vi "SetData.vi"(8 "error in (no error)":errorcluster caption="Fehler (Eingang, kein Fehler)", 9 "Data":variant, 10 "Key":string, 11 "Dictionary Eingang":refnum<class "Dictionary.lvclass"> caption="DNL_LabVIEW Object in") -> (0 "error out":errorcluster caption="Fehler (Ausgang)", 3 "Dictionary Ausgang":refnum<class "Dictionary.lvclass"> caption="DNL_LabVIEW Object out")   [LabVIEW 2013, in "Dictionary.lvclass"]
uses:
  Dictionary.lvclass
  Dictionary.lvclass/Dictionary.ctl
  Properties/GetDict.vi
  Properties/SetDict.vi
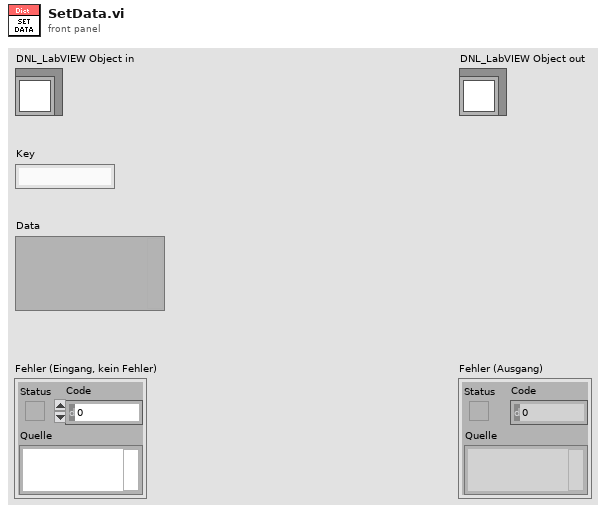
[diagram p1: front panel]
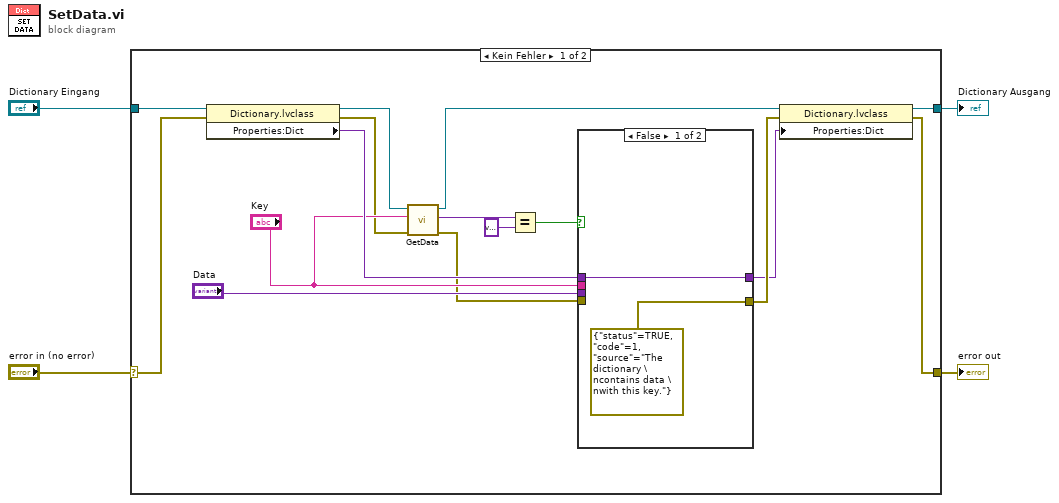
[diagram p0: block diagram]
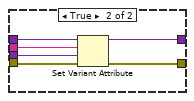
[diagram p2: hidden frame]
diagram:
  n1 = case shown="Kein Fehler" "error in (no error)" {
    selector: "error in (no error)" -> [w13 w30]
    tunnel: [w18 w30] -> w3
    tunnel: [w19 w29] -> w1
    tunnel: "Dictionary Eingang" -> [w20 w29]
    frame No Error {
      n2 = property class="Dictionary.lvclass"(reference=w20, error in=w13) -> (reference out=w12:refnum<class "Dictionary.lvclass">, error out=w10:errorcluster, "Properties:Dict"=w15:variant)
      n3 = call-dynamic "GetData.vi"("error in (no error)"=w10, "Name"="Key", "Dictionary Eingang"=w12) -> ("error out"=w9:errorcluster, "Wert"=w7:variant, "Dictionary Ausgang"=w8:refnum<class "Dictionary.lvclass">)  [unwired: 6 in]
      n4 = Equal?(x=w7, y=variant) -> (x = y?=w5:bool)
      n5 = case shown="False" w5 {
        tunnel: [errorcluster {"status"=TRUE, "code"=1, "source"="The dictionary \ncontains data \nwith this key."} ("error out") w28] -> w17
        tunnel: [w22 w27] -> w16
        tunnel: w15 -> [w22 w26]
        tunnel: "Data" -> [_ w25]
        tunnel: "Key" -> [_ w24]
        tunnel: w9 -> [_ w23]
        frame False {
        }
        frame True {
          n6 = Set Variant Attribute(Variant=w26, name=w24, value=w25, error in=w23) -> (Variant out=w27:variant, error out=w28:errorcluster)  [unwired: 1 out]
        }
      }
      n7 = property class="Dictionary.lvclass"(reference=w8, error in=w17, "Properties:Dict"=w16) -> (reference out=w19:refnum<class "Dictionary.lvclass">, error out=w18:errorcluster)
    }
    frame Error {
    }
  }
  "error out" <- w3
  "Dictionary Ausgang" <- w1
